vi "Detect if NaN.vi"(11 "mean in":dbl) -> (3 "mean out":dbl)   [LabVIEW 2017]
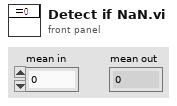
[diagram p1: front panel]
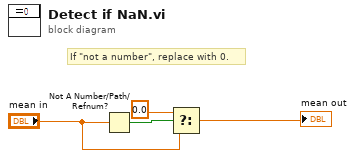
[diagram p0: block diagram]
diagram:
  # "If \"not a number\", replace with 0."
  n1 = Not A Number/Path/Refnum?(number/path/refnum="mean in") -> (NaN/Path/Refnum?=w1:bool)
  n2 = Select(t=0.0, s=w1, f="mean in") -> (s? t:f=→"mean out":dbl)
